vi "SamplesToDisplay-Algo.vi"(6 "InputData":dbl[](array[numeric]), 8 "error in (no error)":errorcluster, 10 "LoopCount":i32, 11 "SamplesToDisplay":i32) -> (0 "error out":errorcluster, 2 "ReducedOutputData":dbl[](array[numeric]))   [LabVIEW 2019, in "Zen Analytics.lvlib" / "Zen Analytics.lvclass"]
uses:
  Zen Analytics.lvclass
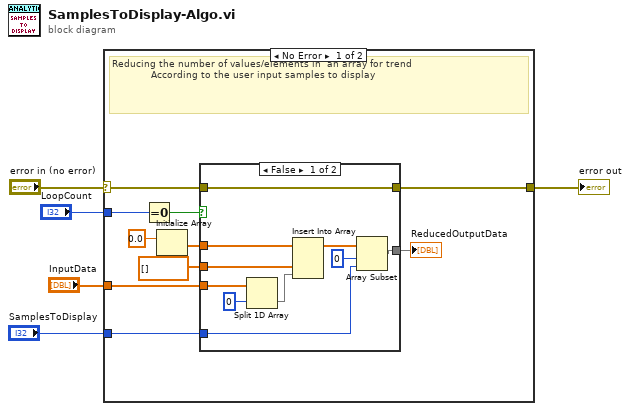
[diagram p0: block diagram]
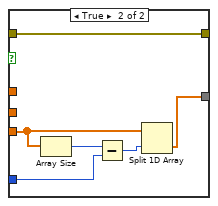
[diagram p2: hidden frame]
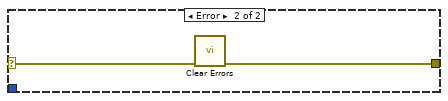
[diagram p3: hidden frame]
diagram:
  n1 = case shown="No Error" "error in (no error)" {
    selector: "error in (no error)" -> [w11 w33]
    tunnel: "SamplesToDisplay" -> [w13 _]
    tunnel: "InputData" -> [w12 _]
    tunnel: [w10 w32] -> w1
    tunnel: "LoopCount" -> [w8 _]
    frame No Error {
      # "Reducing the number of values/elements in  an array for trend\n             According to the user input samples to display"
      n2 = Equal To 0?(x=w8) -> (x = 0?=w7:bool)
      n3 = Initialize Array(0.0 ("element")) -> (w14:dbl[])  [unwired: 1 in]
      n4 = case shown="False" w7 {
        tunnel: w13 -> [w19 w31]
        tunnel: [w18 w28] -> w6
        tunnel: w14 -> [w23 _]
        tunnel: w12 -> [w24 w27]
        tunnel: dbl[] [] -> [w22 _]
        tunnel: w11 -> [w17 w26]
        tunnel: [w17 w26] -> w10
        frame False {
          n5 = Split 1D Array(array=w24, index=0) -> (second subarray=w21:dbl[])  [unwired: 1 out]
          n6 = Insert Into Array(array=w23, new element #1=w22, new element #2=w21) -> (w20:dbl[])  [unwired: 1 in]
          n7 = Array Subset(array=w20, index=0, length=w19) -> (w18:dbl[])
        }
        frame True {
          n8 = Array Size(array=w27) -> (size(s)=w30:i32)
          n9 = Subtract(x=w30, y=w31) -> (x-y=w29:i32)
          n10 = Split 1D Array(array=w27, index=w29) -> (second subarray=w28:dbl[])  [unwired: 1 out]
        }
      }
      "ReducedOutputData" <- w6
    }
    frame Error {
      n11 = call <vilib>:"Clear Errors.vi"("error in (no error)"=w33) -> ("error out"=w32:errorcluster)  [unwired: 5 in, 1 out]
    }
  }
  "error out" <- w1
